vi "Cycle Diag Table Read.vi"(5 "Raw Data In":string) -> (4 "output cluster":T1)   [LabVIEW 2016, in "TLMB.lvlib"]
uses:
  Projects/TLMB.lvlib
  type defs/Cycle_Diag_Teststand.ctl
panel:
  out "appended array":string[](array[string])
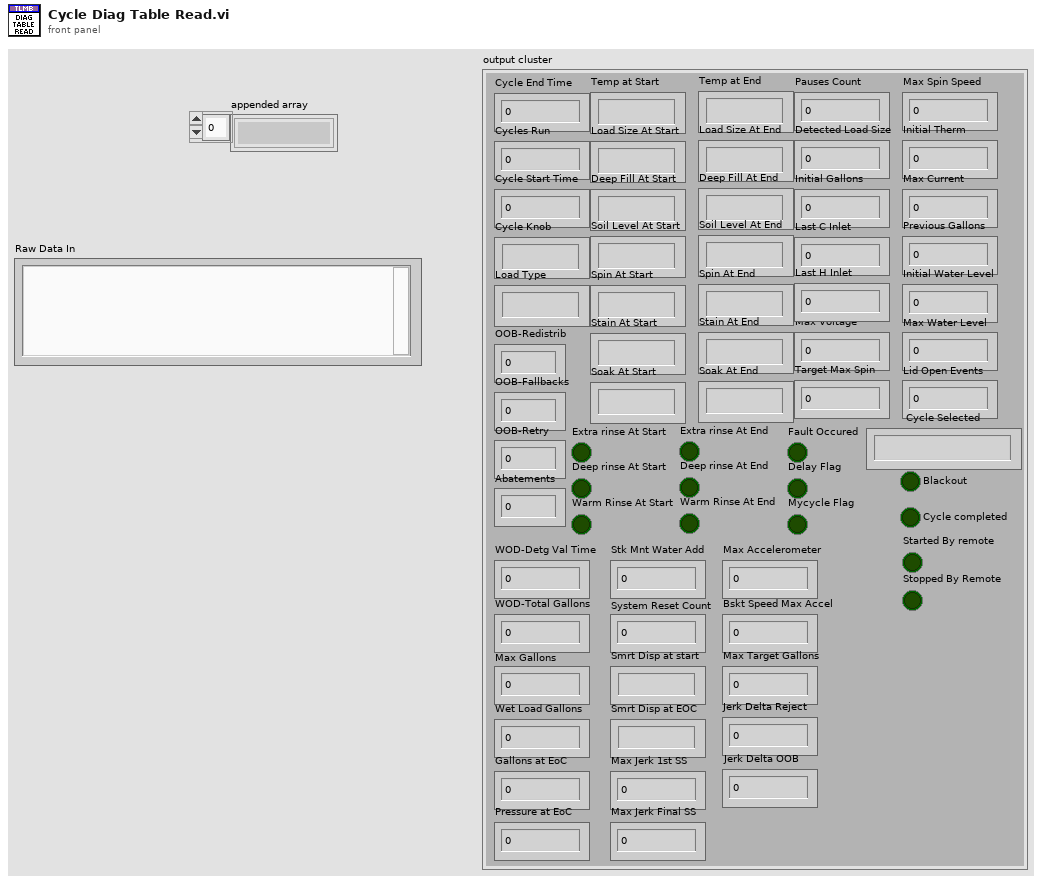
[diagram p1: front panel]
types:
  T1 = typedef "TLMB.lvlib/Cycle_Diag_Teststand.ctl" = cluster{"Cycle End Time":u32, "Cycles Run":u32, "Cycle Start Time":u32, "Cycle Knob":string, "Load Type":string, "OOB-Redistrib":u8, "OOB-Fallbacks":u8, "OOB-Retry":u8, "Temp at Start":string, "Load Size At Start":string, "Deep Fill At Start":string, "Soil Level At Start":string, "Spin At Start":string, "Extra rinse At Start":bool, "Deep rinse At Start":bool, "Stain At Start":string, "Soak At Start":string, "Warm Rinse At Start":bool, "Temp at End":string, "Load Size At End":string, "Deep Fill At End":string, "Soil Level At End":string, "Spin At End":string, "Extra rinse At End":bool, "Deep rinse At End":bool, "Stain At End":string, "Soak At End":string, "Warm Rinse At End":bool, "Pauses Count":u8, "Fault Occured":bool, "Delay Flag":bool, "Mycycle Flag":bool, "Blackout":bool, "Cycle completed":bool, "Detected Load Size":dbl, "Initial Gallons":dbl, "Last C Inlet ":dbl, "Max Voltage":dbl, "Target Max Spin":u16, "Max Spin Speed":u16, "Initial Therm":dbl, "Max Current":dbl, "Previous Gallons":dbl, "Initial Water Level":dbl, "Max Water Level":dbl, "Abatements ":u8, "Lid Open Events":u8, "Cycle Selected":string, "Last H Inlet ":dbl, "WOD-Detg Val Time":u8, "WOD-Total Gallons":u16, "Max Gallons":u16, "Wet Load Gallons":u16, "Gallons at EoC":u16, "Pressure at EoC":u32, "Stk Mnt Water Add":u8, "Started By remote":bool, "Stopped By Remote":bool, "System Reset Count":u8, "Smrt Disp at start":string, "Smrt Disp at EOC":string, "Max Jerk 1st SS":i32, "Max Jerk Final SS":i32, "Max Accelerometer":i16, "Bskt Speed Max Accel":u16, "Max Target Gallons":u16, "Jerk Delta Reject":u8, "Jerk Delta OOB ":u8}
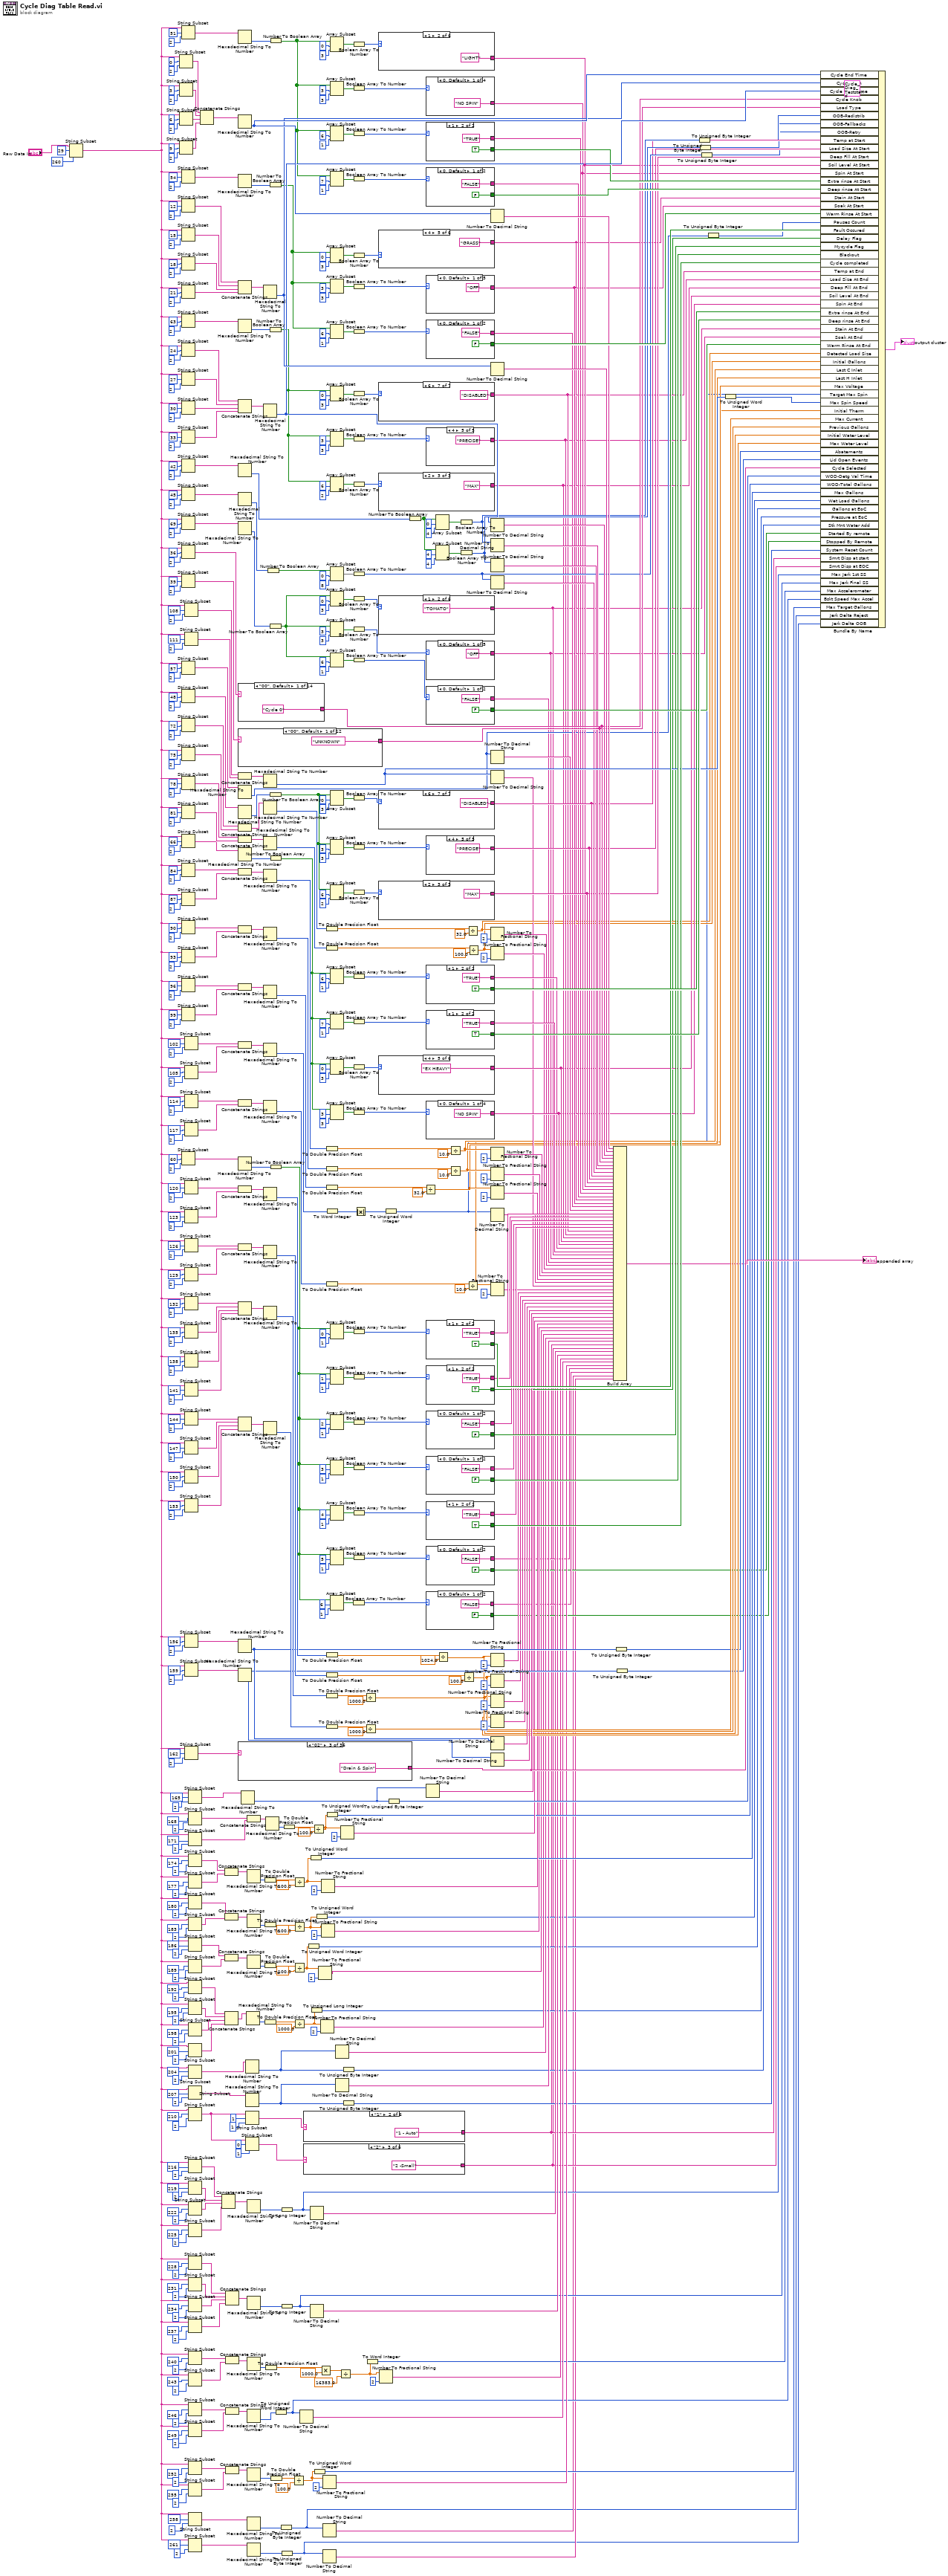
[diagram p0: block diagram]
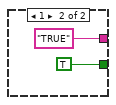
[diagram p2: hidden frame]
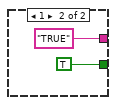
[diagram p3: hidden frame]
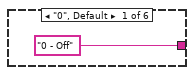
[diagram p4: hidden frame]
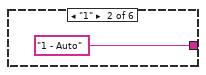
[diagram p5: hidden frame]
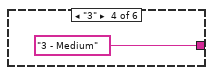
[diagram p6: hidden frame]
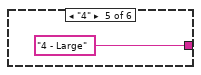
[diagram p7: hidden frame]
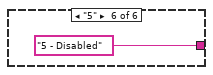
[diagram p8: hidden frame]
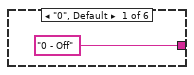
[diagram p9: hidden frame]
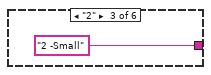
[diagram p10: hidden frame]
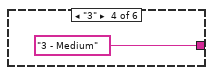
[diagram p11: hidden frame]
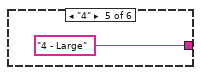
[diagram p12: hidden frame]
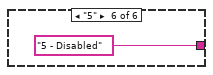
[diagram p13: hidden frame]
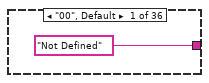
[diagram p14: hidden frame]
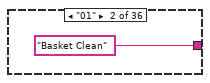
[diagram p15: hidden frame]
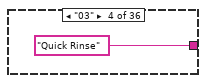
[diagram p16: hidden frame]
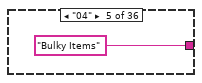
[diagram p17: hidden frame]
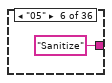
[diagram p18: hidden frame]
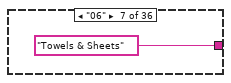
[diagram p19: hidden frame]
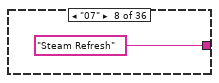
[diagram p20: hidden frame]
diagram:
  n1 = String Subset(string="Raw Data In", offset (0)=29, length (rest)=260 ("length (rest)")) -> (substring=w13:string)
  n2 = String Subset(string=w13, offset (0)=0, length (rest)=2 ("length (rest)")) -> (substring=w614:string)
  n3 = String Subset(string=w13, offset (0)=3, length (rest)=2 ("length (rest)")) -> (substring=w613:string)
  n4 = String Subset(string=w13, offset (0)=6, length (rest)=2 ("length (rest)")) -> (substring=w612:string)
  n5 = String Subset(string=w13, offset (0)=9, length (rest)=2 ("length (rest)")) -> (substring=w611:string)
  n6 = String Subset(string=w13, offset (0)=51, length (rest)=2 ("length (rest)")) -> (substring=w317:string)
  n7 = String Subset(string=w13, offset (0)=54, length (rest)=2 ("length (rest)")) -> (substring=w301:string)
  n8 = String Subset(string=w13, offset (0)=12, length (rest)=2 ("length (rest)")) -> (substring=w608:string)
  n9 = String Subset(string=w13, offset (0)=15, length (rest)=2 ("length (rest)")) -> (substring=w607:string)
  n10 = String Subset(string=w13, offset (0)=18, length (rest)=2 ("length (rest)")) -> (substring=w606:string)
  n11 = String Subset(string=w13, offset (0)=21, length (rest)=2 ("length (rest)")) -> (substring=w605:string)
  n12 = String Subset(string=w13, offset (0)=63, length (rest)=2 ("length (rest)")) -> (substring=w288:string)
  n13 = String Subset(string=w13, offset (0)=24, length (rest)=2 ("length (rest)")) -> (substring=w602:string)
  n14 = String Subset(string=w13, offset (0)=27, length (rest)=2 ("length (rest)")) -> (substring=w601:string)
  n15 = String Subset(string=w13, offset (0)=30, length (rest)=2 ("length (rest)")) -> (substring=w600:string)
  n16 = String Subset(string=w13, offset (0)=33, length (rest)=2 ("length (rest)")) -> (substring=w599:string)
  n17 = String Subset(string=w13, offset (0)=42, length (rest)=2 ("length (rest)")) -> (substring=w257:string)
  n18 = String Subset(string=w13, offset (0)=45, length (rest)=2 ("length (rest)")) -> (substring=w248:string)
  n19 = String Subset(string=w13, offset (0)=69, length (rest)=2 ("length (rest)")) -> (substring=w261:string)
  n20 = String Subset(string=w13, offset (0)=36, length (rest)=2 ("length (rest)")) -> (substring=w596:string)
  n21 = String Subset(string=w13, offset (0)=39, length (rest)=2 ("length (rest)")) -> (substring=w595:string)
  n22 = String Subset(string=w13, offset (0)=57, length (rest)=2 ("length (rest)")) -> (substring=w553:string)
  n23 = String Subset(string=w13, offset (0)=48, length (rest)=2 ("length (rest)")) -> (substring=w336:string)
  n24 = String Subset(string=w13, offset (0)=72, length (rest)=2 ("length (rest)")) -> (substring=w537:string)
  n25 = String Subset(string=w13, offset (0)=75 ("offset"), length (rest)=u32 2 ("default (0 U32)")) -> (substring=w534:string)
  n26 = String Subset(string=w13, offset (0)=78, length (rest)=2 ("length (rest)")) -> (substring=w529:string)
  n27 = String Subset(string=w13, offset (0)=81, length (rest)=2 ("length (rest)")) -> (substring=w528:string)
  n28 = String Subset(string=w13, offset (0)=66, length (rest)=2 ("length (rest)")) -> (substring=w274:string)
  n29 = String Subset(string=w13, offset (0)=84, length (rest)=2 ("length (rest)")) -> (substring=w518:string)
  n30 = String Subset(string=w13, offset (0)=87, length (rest)=2 ("length (rest)")) -> (substring=w517:string)
  n31 = String Subset(string=w13, offset (0)=90, length (rest)=2 ("length (rest)")) -> (substring=w512:string)
  n32 = String Subset(string=w13, offset (0)=93, length (rest)=2 ("length (rest)")) -> (substring=w511:string)
  n33 = String Subset(string=w13, offset (0)=96, length (rest)=2 ("length (rest)")) -> (substring=w502:string)
  n34 = String Subset(string=w13, offset (0)=99, length (rest)=2 ("length (rest)")) -> (substring=w501:string)
  n35 = String Subset(string=w13, offset (0)=60, length (rest)=2 ("length (rest)")) -> (substring=w552:string)
  n36 = String Subset(string=w13, offset (0)=108, length (rest)=2 ("length (rest)")) -> (substring=w489:string)
  n37 = String Subset(string=w13, offset (0)=111, length (rest)=2 ("length (rest)")) -> (substring=w488:string)
  n38 = String Subset(string=w13, offset (0)=102, length (rest)=2 ("length (rest)")) -> (substring=w492:string)
  n39 = String Subset(string=w13, offset (0)=105, length (rest)=2 ("length (rest)")) -> (substring=w491:string)
  n40 = String Subset(string=w13, offset (0)=114, length (rest)=2 ("length (rest)")) -> (substring=w477:string)
  n41 = String Subset(string=w13, offset (0)=117, length (rest)=2 ("length (rest)")) -> (substring=w476:string)
  n42 = String Subset(string=w13, offset (0)=120, length (rest)=2 ("length (rest)")) -> (substring=w467:string)
  n43 = String Subset(string=w13, offset (0)=123, length (rest)=2 ("length (rest)")) -> (substring=w466:string)
  n44 = String Subset(string=w13, offset (0)=126, length (rest)=2 ("length (rest)")) -> (substring=w457:string)
  n45 = String Subset(string=w13, offset (0)=129, length (rest)=2 ("length (rest)")) -> (substring=w456:string)
  n46 = String Subset(string=w13, offset (0)=132, length (rest)=2 ("length (rest)")) -> (substring=w447:string)
  n47 = String Subset(string=w13, offset (0)=135, length (rest)=2 ("length (rest)")) -> (substring=w446:string)
  n48 = String Subset(string=w13, offset (0)=138, length (rest)=2 ("length (rest)")) -> (substring=w416:string)
  n49 = String Subset(string=w13, offset (0)=141, length (rest)=2 ("length (rest)")) -> (substring=w415:string)
  n50 = String Subset(string=w13, offset (0)=144, length (rest)=2 ("length (rest)")) -> (substring=w441:string)
  n51 = String Subset(string=w13, offset (0)=147, length (rest)=2 ("length (rest)")) -> (substring=w440:string)
  n52 = String Subset(string=w13, offset (0)=150, length (rest)=2 ("length (rest)")) -> (substring=w410:string)
  n53 = String Subset(string=w13, offset (0)=153, length (rest)=2 ("length (rest)")) -> (substring=w409:string)
  n54 = String Subset(string=w13, offset (0)=156, length (rest)=2 ("length (rest)")) -> (substring=w421:string)
  n55 = String Subset(string=w13, offset (0)=159, length (rest)=2 ("length (rest)")) -> (substring=w420:string)
  n56 = String Subset(string=w13, offset (0)=162, length (rest)=2 ("length (rest)")) -> (substring=w417:string)
  n57 = String Subset(string=w13, offset (0)=165 ("length (rest)"), length (rest)=2 ("length (rest)")) -> (substring=w143:string)
  n58 = String Subset(string=w13, offset (0)=168 ("length (rest)"), length (rest)=2 ("length (rest)")) -> (substring=w141:string)
  n59 = String Subset(string=w13, offset (0)=171 ("length (rest)"), length (rest)=2 ("length (rest)")) -> (substring=w140:string)
  n60 = String Subset(string=w13, offset (0)=174 ("length (rest)"), length (rest)=2 ("length (rest)")) -> (substring=w131:string)
  n61 = String Subset(string=w13, offset (0)=177 ("length (rest)"), length (rest)=2 ("length (rest)")) -> (substring=w130:string)
  n62 = String Subset(string=w13, offset (0)=180 ("length (rest)"), length (rest)=2 ("length (rest)")) -> (substring=w121:string)
  n63 = String Subset(string=w13, offset (0)=183 ("length (rest)"), length (rest)=2 ("length (rest)")) -> (substring=w120:string)
  n64 = String Subset(string=w13, offset (0)=186 ("length (rest)"), length (rest)=2 ("length (rest)")) -> (substring=w119:string)
  n65 = String Subset(string=w13, offset (0)=189 ("length (rest)"), length (rest)=2 ("length (rest)")) -> (substring=w118:string)
  n66 = String Subset(string=w13, offset (0)=192 ("length (rest)"), length (rest)=2 ("length (rest)")) -> (substring=w117:string)
  n67 = String Subset(string=w13, offset (0)=195 ("length (rest)"), length (rest)=2 ("length (rest)")) -> (substring=w116:string)
  n68 = String Subset(string=w13, offset (0)=198 ("length (rest)"), length (rest)=2 ("length (rest)")) -> (substring=w115:string)
  n69 = String Subset(string=w13, offset (0)=201 ("length (rest)"), length (rest)=2 ("length (rest)")) -> (substring=w114:string)
  n70 = String Subset(string=w13, offset (0)=204 ("length (rest)"), length (rest)=2 ("length (rest)")) -> (substring=w109:string)
  n71 = String Subset(string=w13, offset (0)=207 ("length (rest)"), length (rest)=2 ("length (rest)")) -> (substring=w106:string)
  n72 = String Subset(string=w13, offset (0)=210 ("length (rest)"), length (rest)=2 ("length (rest)")) -> (substring=w105:string)
  n73 = String Subset(string=w13, offset (0)=216 ("length (rest)"), length (rest)=2 ("length (rest)")) -> (substring=w98:string)
  n74 = String Subset(string=w13, offset (0)=219 ("length (rest)"), length (rest)=2 ("length (rest)")) -> (substring=w97:string)
  n75 = String Subset(string=w13, offset (0)=222 ("length (rest)"), length (rest)=2 ("length (rest)")) -> (substring=w96:string)
  n76 = String Subset(string=w13, offset (0)=225 ("length (rest)"), length (rest)=2 ("length (rest)")) -> (substring=w95:string)
  n77 = String Subset(string=w13, offset (0)=228 ("length (rest)"), length (rest)=2 ("length (rest)")) -> (substring=w92:string)
  n78 = String Subset(string=w13, offset (0)=231 ("length (rest)"), length (rest)=2 ("length (rest)")) -> (substring=w91:string)
  n79 = String Subset(string=w13, offset (0)=234 ("length (rest)"), length (rest)=2 ("length (rest)")) -> (substring=w90:string)
  n80 = String Subset(string=w13, offset (0)=237 ("length (rest)"), length (rest)=2 ("length (rest)")) -> (substring=w89:string)
  n81 = String Subset(string=w13, offset (0)=240 ("length (rest)"), length (rest)=2 ("length (rest)")) -> (substring=w86:string)
  n82 = String Subset(string=w13, offset (0)=243 ("length (rest)"), length (rest)=2 ("length (rest)")) -> (substring=w85:string)
  n83 = String Subset(string=w13, offset (0)=246 ("length (rest)"), length (rest)=2 ("length (rest)")) -> (substring=w84:string)
  n84 = String Subset(string=w13, offset (0)=249 ("length (rest)"), length (rest)=2 ("length (rest)")) -> (substring=w83:string)
  n85 = String Subset(string=w13, offset (0)=252 ("length (rest)"), length (rest)=2 ("length (rest)")) -> (substring=w82:string)
  n86 = String Subset(string=w13, offset (0)=255 ("length (rest)"), length (rest)=2 ("length (rest)")) -> (substring=w81:string)
  n87 = String Subset(string=w13, offset (0)=258, length (rest)=2 ("length (rest)")) -> (substring=w8:string)
  n88 = String Subset(string=w13, offset (0)=261, length (rest)=2 ("length (rest)")) -> (substring=w7:string)
  n89 = Concatenate Strings(w614, w613, w612, w611) -> (w610:string)
  n90 = Concatenate Strings(w98, w97, w96, w95) -> (w94:string)
  n91 = Concatenate Strings(w131, w130) -> (w135:string)
  n92 = Concatenate Strings(w121, w120) -> (w129:string)
  n93 = Concatenate Strings(w119, w118) -> (w125:string)
  n94 = Concatenate Strings(w117, w116, w115, w114) -> (w110:string)
  n95 = Concatenate Strings(w92, w91, w90, w89) -> (w88:string)
  n96 = Concatenate Strings(w86, w85) -> (w79:string)
  n97 = Concatenate Strings(w84, w83) -> (w74:string)
  n98 = Concatenate Strings(w82, w81) -> (w72:string)
  n99 = Hexadecimal String To Number(string=w317) -> (number=w324:u32)  [unwired: 2 in, 1 out]
  n100 = Hexadecimal String To Number(string=w610) -> (number=w609:u32)  [unwired: 2 in, 1 out]
  n101 = Hexadecimal String To Number(string=w301) -> (number=w309:u32)  [unwired: 2 in, 1 out]
  n102 = Concatenate Strings(w608, w607, w606, w605) -> (w604:string)
  n103 = Hexadecimal String To Number(string=w288) -> (number=w296:u32)  [unwired: 2 in, 1 out]
  n104 = Concatenate Strings(w602, w601, w600, w599) -> (w598:string)
  n105 = Hexadecimal String To Number(string=w257) -> (number=w256:u32)  [unwired: 2 in, 1 out]
  n106 = Hexadecimal String To Number(string=w248) -> (number=w247:u32)  [unwired: 2 in, 1 out]
  n107 = Hexadecimal String To Number(string=w261) -> (number=w269:u32)  [unwired: 2 in, 1 out]
  n108 = case shown="\"00\", Default" w596 {
    tunnel: ["Cycle 0" "Cycle 1" "Cycle 2" "Cycle 3" "Cycle 4" "Cycle 5" "Cycle 6" "Cycle 7" "Cycle 8" "Cycle 9" "Cycle 10" "Cycle 11" "Cycle 12" "Cycle 13"] -> w397
    frame "00", Default {
    }
    frame "01" {
    }
    frame "02" {
    }
    frame "03" {
    }
    frame "04" {
    }
    frame "05" {
    }
    frame "06" {
    }
    frame "07" {
    }
    frame "08" {
    }
    frame "09" {
    }
    frame "0A" {
    }
    frame "0B" {
    }
    frame "0C" {
    }
    frame "0D" {
    }
  }
  n109 = case shown="\"00\", Default" w595 {
    tunnel: ["UNKNOWN" "COTTON" "SYNTHETIC" "MIXED" "WET" "LOW FLOW" "SMALL" "MEDIUM" "LARGE" "SUPER" "SUPER PLUS" "MAX"] -> w396
    frame "00", Default {
    }
    frame "01" {
    }
    frame "02" {
    }
    frame "03" {
    }
    frame "04" {
    }
    frame "05" {
    }
    frame "06" {
    }
    frame "07" {
    }
    frame "08" {
    }
    frame "09" {
    }
    frame "0A" {
    }
    frame "0B" {
    }
  }
  n110 = Concatenate Strings(w489, w488) -> (w487:string)
  n111 = Hexadecimal String To Number(string=w553) -> (number=w380:u32)  [unwired: 2 in, 1 out]
  n112 = Hexadecimal String To Number(string=w336) -> (number=w335:u32)  [unwired: 2 in, 1 out]
  n113 = Concatenate Strings(w537, w534) -> (w533:string)
  n114 = Concatenate Strings(w529, w528) -> (w527:string)
  n115 = Hexadecimal String To Number(string=w274) -> (number=w284:u32)  [unwired: 2 in, 1 out]
  n116 = Concatenate Strings(w518, w517) -> (w516:string)
  n117 = Concatenate Strings(w512, w511) -> (w510:string)
  n118 = Concatenate Strings(w502, w501) -> (w500:string)
  n119 = Concatenate Strings(w492, w491) -> (w490:string)
  n120 = Concatenate Strings(w477, w476) -> (w475:string)
  n121 = Hexadecimal String To Number(string=w552) -> (number=w551:u32)  [unwired: 2 in, 1 out]
  n122 = Concatenate Strings(w467, w466) -> (w465:string)
  n123 = Concatenate Strings(w457, w456) -> (w455:string)
  n124 = Concatenate Strings(w447, w446, w416, w415) -> (w445:string)
  n125 = Concatenate Strings(w441, w440, w410, w409) -> (w439:string)
  n126 = Hexadecimal String To Number(string=w421) -> (number=w419:u32)  [unwired: 2 in, 1 out]
  n127 = Hexadecimal String To Number(string=w420) -> (number=w418:u32)  [unwired: 2 in, 1 out]
  n128 = case shown="\"02\"" w417 {
    tunnel: ["Not Defined" "Basket Clean" "Drain & Spin" "Quick Rinse" "Bulky Items" "Sanitize" "Towels & Sheets" "Steam Refresh" "Normal/Mixed" "Whites" "Dark Colors" "Jeans" "Hand Wash" "Delicates" "Speed Wash" "Heavy Duty" "Allergen" "Power Clean" "Rinse & Spin" "Single Item" "Colors" "Cold Wash" "Cottons" "Easy Care" "Active Wear" "Timed Dry" "Dewrinkle" "Air Fluff" "Steam Refresh" "Steam Dewrinkle" "Speed Dry" "Mixed" "Quick Dry" "Casuals" "Warm Up" "Energy Saver"] -> w347
    frame "00", Default {
    }
    frame "01" {
    }
    frame "02" {
    }
    frame "03" {
    }
    frame "04" {
    }
    frame "05" {
    }
    frame "06" {
    }
    frame "07" {
    }
    frame "08" {
    }
    frame "09" {
    }
    frame "0A" {
    }
    frame "0B" {
    }
    frame "0C" {
    }
    frame "0D" {
    }
    frame "0E" {
    }
    frame "0F" {
    }
    frame "10" {
    }
    frame "11" {
    }
    frame "12" {
    }
    frame "13" {
    }
    frame "14" {
    }
    frame "15" {
    }
    frame "80" {
    }
    frame "81" {
    }
    frame "82" {
    }
    frame "83" {
    }
    frame "84" {
    }
    frame "85" {
    }
    frame "86" {
    }
    frame "87" {
    }
    frame "88" {
    }
    frame "89" {
    }
    frame "8A" {
    }
    frame "8B" {
    }
    frame "8C" {
    }
    frame "8D" {
    }
  }
  n129 = Hexadecimal String To Number(string=w143) -> (number=w142:u32)  [unwired: 2 in, 1 out]
  n130 = Hexadecimal String To Number(string=w109) -> (number=w108:u32)  [unwired: 2 in, 1 out]
  n131 = Hexadecimal String To Number(string=w106) -> (number=w107:u32)  [unwired: 2 in, 1 out]
  n132 = String Subset(string=w105, offset (0)=1, length (rest)=1 ("length (rest)")) -> (substring=w100:string)
  n133 = String Subset(string=w105, offset (0)=0, length (rest)=1 ("length (rest)")) -> (substring=w99:string)
  n134 = Hexadecimal String To Number(string=w110) -> (number=w113:u32)  [unwired: 2 in, 1 out]
  n135 = Concatenate Strings(w141, w140) -> (w139:string)
  n136 = Hexadecimal String To Number(string=w135) -> (number=w134:u32)  [unwired: 2 in, 1 out]
  n137 = Hexadecimal String To Number(string=w129) -> (number=w128:u32)  [unwired: 2 in, 1 out]
  n138 = Hexadecimal String To Number(string=w125) -> (number=w124:u32)  [unwired: 2 in, 1 out]
  n139 = Hexadecimal String To Number(string=w79) -> (number=w80:u32)  [unwired: 2 in, 1 out]
  n140 = Hexadecimal String To Number(string=w74) -> (number=w55:u32)  [unwired: 2 in, 1 out]
  n141 = Hexadecimal String To Number(string=w72) -> (number=w73:u32)  [unwired: 2 in, 1 out]
  n142 = Hexadecimal String To Number(string=w8) -> (number=w6:u32)  [unwired: 2 in, 1 out]
  n143 = Hexadecimal String To Number(string=w7) -> (number=w5:u32)  [unwired: 2 in, 1 out]
  n144 = Hexadecimal String To Number(string=w94) -> (number=w93:u32)  [unwired: 2 in, 1 out]
  n145 = Hexadecimal String To Number(string=w88) -> (number=w87:u32)  [unwired: 2 in, 1 out]
  n146 = Hexadecimal String To Number(string=w604) -> (number=w603:u32)  [unwired: 2 in, 1 out]
  n147 = Hexadecimal String To Number(string=w598) -> (number=w597:u32)  [unwired: 2 in, 1 out]
  n148 = Hexadecimal String To Number(string=w487) -> (number=w486:u32)  [unwired: 2 in, 1 out]
  n149 = Hexadecimal String To Number(string=w533) -> (number=w540:u32)  [unwired: 2 in, 1 out]
  n150 = Hexadecimal String To Number(string=w527) -> (number=w526:u32)  [unwired: 2 in, 1 out]
  n151 = Hexadecimal String To Number(string=w516) -> (number=w515:u32)  [unwired: 2 in, 1 out]
  n152 = Hexadecimal String To Number(string=w510) -> (number=w509:u32)  [unwired: 2 in, 1 out]
  n153 = Hexadecimal String To Number(string=w500) -> (number=w499:u32)  [unwired: 2 in, 1 out]
  n154 = Hexadecimal String To Number(string=w490) -> (number=w402:u32)  [unwired: 2 in, 1 out]
  n155 = Hexadecimal String To Number(string=w475) -> (number=w474:u32)  [unwired: 2 in, 1 out]
  n156 = Hexadecimal String To Number(string=w465) -> (number=w464:u32)  [unwired: 2 in, 1 out]
  n157 = Hexadecimal String To Number(string=w455) -> (number=w454:u32)  [unwired: 2 in, 1 out]
  n158 = Hexadecimal String To Number(string=w445) -> (number=w444:u32)  [unwired: 2 in, 1 out]
  n159 = Hexadecimal String To Number(string=w439) -> (number=w438:u32)  [unwired: 2 in, 1 out]
  n160 = To Double Precision Float(number=w134) -> (double precision float=w133:dbl)
  n161 = To Double Precision Float(number=w128) -> (double precision float=w127:dbl)
  n162 = To Double Precision Float(number=w124) -> (double precision float=w123:dbl)
  n163 = To Double Precision Float(number=w113) -> (double precision float=w112:dbl)
  n164 = To Double Precision Float(number=w80) -> (double precision float=w78:dbl)
  n165 = Hexadecimal String To Number(string=w139) -> (number=w138:u32)  [unwired: 2 in, 1 out]
  n166 = Number To Boolean Array(number=w247) -> (Boolean array=w246:bool[])
  n167 = Number To Boolean Array(number=w309) -> (Boolean array=w308:bool[])
  n168 = Number To Boolean Array(number=w296) -> (Boolean array=w295:bool[])
  n169 = Number To Boolean Array(number=w269) -> (Boolean array=w268:bool[])
  n170 = Number To Boolean Array(number=w335) -> (Boolean array=w334:bool[])
  n171 = Number To Boolean Array(number=w324) -> (Boolean array=w316:bool[])
  n172 = Number To Boolean Array(number=w284) -> (Boolean array=w277:bool[])
  n173 = Number To Boolean Array(number=w551) -> (Boolean array=w30:bool[])
  n174 = To Double Precision Float(number=w73) -> (double precision float=w71:dbl)
  n175 = To Unsigned Word Integer(number=w55) -> (unsigned 16bit integer=w15:u16)
  n176 = To Unsigned Byte Integer(number=w6) -> (unsigned 8bit integer=w2:u8)
  n177 = To Long Integer(number=w93) -> (32bit integer=w18:i32)
  n178 = To Long Integer(number=w87) -> (32bit integer=w17:i32)
  n179 = To Unsigned Byte Integer(number=w5) -> (unsigned 8bit integer=w1:u8)
  n180 = To Double Precision Float(number=w138) -> (double precision float=w137:dbl)
  n181 = Divide(x=w71, y=100.0) -> (x/y=w63:dbl)
  n182 = Divide(x=w133, y=100.0) -> (x/y=w68:dbl)
  n183 = Divide(x=w127, y=100.0) -> (x/y=w67:dbl)
  n184 = Divide(x=w123, y=100.0) -> (x/y=w66:dbl)
  n185 = Divide(x=w112, y=1000.0) -> (x/y=w65:dbl)
  n186 = Number To Decimal String(number=w15) -> (decimal integer string=w40:string)  [unwired: 1 in]
  n187 = case shown="\"2\"" w99 {
    tunnel: ["0 - Off" "1 - Auto" "2 -Small" "3 - Medium" "4 - Large" "5 - Disabled"] -> w19
    frame "0", Default {
    }
    frame "1" {
    }
    frame "2" {
    }
    frame "3" {
    }
    frame "4" {
    }
    frame "5" {
    }
  }
  n188 = case shown="\"1\"" w100 {
    tunnel: ["0 - Off" "1 - Auto" "2 -Small" "3 - Medium" "4 - Large" "5 - Disabled"] -> w20
    frame "0", Default {
    }
    frame "1" {
    }
    frame "2" {
    }
    frame "3" {
    }
    frame "4" {
    }
    frame "5" {
    }
  }
  n189 = To Unsigned Word Integer(number=w66) -> (unsigned 16bit integer=w26:u16)
  n190 = To Unsigned Word Integer(number=w68) -> (unsigned 16bit integer=w49:u16)
  n191 = To Unsigned Long Integer(number=w65) -> (unsigned 32bit integer=w25:u32)
  n192 = Number To Decimal String(number=w18) -> (decimal integer string=w43:string)  [unwired: 1 in]
  n193 = Number To Decimal String(number=w17) -> (decimal integer string=w42:string)  [unwired: 1 in]
  n194 = Divide(x=w137, y=100.0) -> (x/y=w69:dbl)
  n195 = To Unsigned Word Integer(number=w63) -> (unsigned 16bit integer=w14:u16)
  n196 = To Unsigned Word Integer(number=w67) -> (unsigned 16bit integer=w27:u16)
  n197 = Number To Fractional String(number=w66, precision (6)=i16 2) -> (F-format string=w47:string)  [unwired: 2 in]
  n198 = Multiply(x=w78, y=1000.0) -> (x*y=w76:dbl)
  n199 = Number To Fractional String(number=w65, precision (6)=i16 2) -> (F-format string=w46:string)  [unwired: 2 in]
  n200 = Number To Fractional String(number=w68, precision (6)=i16 2) -> (F-format string=w50:string)  [unwired: 2 in]
  n201 = Number To Fractional String(number=w67, precision (6)=i16 2) -> (F-format string=w48:string)  [unwired: 2 in]
  n202 = Number To Fractional String(number=w63, precision (6)=i16 2) -> (F-format string=w39:string)  [unwired: 2 in]
  n203 = Number To Decimal String(number=w2) -> (decimal integer string=w4:string)  [unwired: 1 in]
  n204 = Number To Decimal String(number=w1) -> (decimal integer string=w3:string)  [unwired: 1 in]
  n205 = To Double Precision Float(number=w540) -> (double precision float=w539:dbl)
  n206 = To Double Precision Float(number=w526) -> (double precision float=w525:dbl)
  n207 = To Double Precision Float(number=w515) -> (double precision float=w514:dbl)
  n208 = To Double Precision Float(number=w509) -> (double precision float=w508:dbl)
  n209 = To Double Precision Float(number=w499) -> (double precision float=w498:dbl)
  n210 = To Word Integer(number=w402) -> (16bit integer=w404:i16)
  n211 = To Double Precision Float(number=w474) -> (double precision float=w473:dbl)
  n212 = To Double Precision Float(number=w464) -> (double precision float=w463:dbl)
  n213 = To Double Precision Float(number=w454) -> (double precision float=w453:dbl)
  n214 = To Double Precision Float(number=w444) -> (double precision float=w443:dbl)
  n215 = To Double Precision Float(number=w438) -> (double precision float=w437:dbl)
  n216 = To Unsigned Word Integer(number=w69) -> (unsigned 16bit integer=w51:u16)
  n217 = Array Subset(array=w30, index=6, length=1) -> (w31:bool[])
  n218 = Array Subset(array=w316, index=0, length=3) -> (w313:bool[])
  n219 = Array Subset(array=w316, index=3, length=3) -> (w312:bool[])
  n220 = Array Subset(array=w316, index=6, length=1) -> (w311:bool[])
  n221 = Array Subset(array=w316, index=7, length=1) -> (w310:bool[])
  n222 = Array Subset(array=w308, index=0, length=3) -> (w299:bool[])
  n223 = Array Subset(array=w308, index=3, length=3) -> (w298:bool[])
  n224 = Array Subset(array=w308, index=6, length=1) -> (w297:bool[])
  n225 = Array Subset(array=w295, index=0, length=3) -> (w287:bool[])
  n226 = Array Subset(array=w295, index=3, length=3) -> (w286:bool[])
  n227 = Array Subset(array=w295, index=6, length=2) -> (w285:bool[])
  n228 = Array Subset(array=w246, index=0, length=8) -> (w243:bool[])
  n229 = Array Subset(array=w268, index=0, length=3) -> (w260:bool[])
  n230 = Array Subset(array=w268, index=3, length=3) -> (w259:bool[])
  n231 = Array Subset(array=w268, index=6, length=1) -> (w258:bool[])
  n232 = Array Subset(array=w334, index=0, length=3) -> (w327:bool[])
  n233 = Array Subset(array=w334, index=3, length=3) -> (w326:bool[])
  n234 = Array Subset(array=w334, index=6, length=2) -> (w325:bool[])
  n235 = Array Subset(array=w277, index=6, length=1) -> (w271:bool[])
  n236 = Array Subset(array=w277, index=7, length=1) -> (w270:bool[])
  n237 = Array Subset(array=w277, index=0, length=3) -> (w273:bool[])
  n238 = Array Subset(array=w277, index=3, length=3) -> (w272:bool[])
  n239 = Array Subset(array=w30, index=0, length=1) -> (w232:bool[])
  n240 = Array Subset(array=w30, index=1, length=1) -> (w230:bool[])
  n241 = Array Subset(array=w30, index=2, length=1) -> (w229:bool[])
  n242 = Array Subset(array=w30, index=3, length=1) -> (w228:bool[])
  n243 = Array Subset(array=w30, index=4, length=1) -> (w227:bool[])
  n244 = Array Subset(array=w30, index=5, length=1) -> (w35:bool[])
  n245 = Number To Decimal String(number=w108) -> (decimal integer string=w45:string)  [unwired: 1 in]
  n246 = Number To Decimal String(number=w107) -> (decimal integer string=w44:string)  [unwired: 1 in]
  n247 = Divide(x=w76, y=16383.0) -> (x/y=w64:dbl)
  n248 = Number To Fractional String(number=w69, precision (6)=i16 2) -> (F-format string=w52:string)  [unwired: 2 in]
  n249 = To Unsigned Byte Integer(number=w108) -> (unsigned 8bit integer=w24:u8)
  n250 = To Unsigned Byte Integer(number=w107) -> (unsigned 8bit integer=w21:u8)
  n251 = Boolean Array To Number(Boolean array=w31) -> (number=w34:u32)
  n252 = Boolean Array To Number(Boolean array=w313) -> (number=w586:u32)
  n253 = Boolean Array To Number(Boolean array=w312) -> (number=w585:u32)
  n254 = Boolean Array To Number(Boolean array=w311) -> (number=w584:u32)
  n255 = Boolean Array To Number(Boolean array=w310) -> (number=w583:u32)
  n256 = Boolean Array To Number(Boolean array=w299) -> (number=w580:u32)
  n257 = Boolean Array To Number(Boolean array=w298) -> (number=w579:u32)
  n258 = Boolean Array To Number(Boolean array=w297) -> (number=w578:u32)
  n259 = Boolean Array To Number(Boolean array=w287) -> (number=w570:u32)
  n260 = Boolean Array To Number(Boolean array=w286) -> (number=w569:u32)
  n261 = Boolean Array To Number(Boolean array=w285) -> (number=w568:u32)
  n262 = Boolean Array To Number(Boolean array=w243) -> (number=w390:u32)
  n263 = Boolean Array To Number(Boolean array=w260) -> (number=w563:u32)
  n264 = Boolean Array To Number(Boolean array=w259) -> (number=w562:u32)
  n265 = Boolean Array To Number(Boolean array=w258) -> (number=w561:u32)
  n266 = Boolean Array To Number(Boolean array=w327) -> (number=w401:u32)
  n267 = Boolean Array To Number(Boolean array=w326) -> (number=w588:u32)
  n268 = Boolean Array To Number(Boolean array=w325) -> (number=w587:u32)
  n269 = Boolean Array To Number(Boolean array=w271) -> (number=w565:u32)
  n270 = Boolean Array To Number(Boolean array=w270) -> (number=w564:u32)
  n271 = Boolean Array To Number(Boolean array=w273) -> (number=w567:u32)
  n272 = Boolean Array To Number(Boolean array=w272) -> (number=w566:u32)
  n273 = Boolean Array To Number(Boolean array=w232) -> (number=w550:u32)
  n274 = Boolean Array To Number(Boolean array=w230) -> (number=w549:u32)
  n275 = Boolean Array To Number(Boolean array=w229) -> (number=w548:u32)
  n276 = Boolean Array To Number(Boolean array=w228) -> (number=w547:u32)
  n277 = Boolean Array To Number(Boolean array=w227) -> (number=w546:u32)
  n278 = Boolean Array To Number(Boolean array=w35) -> (number=w38:u32)
  n279 = Absolute Value(x=w404) -> (abs(x)=w403:i16)
  n280 = Divide(x=w443, y=1000.0) -> (x/y=w340:dbl)
  n281 = Divide(x=w437, y=1000.0) -> (x/y=w339:dbl)
  n282 = To Word Integer(number=w64) -> (16bit integer=w16:i16)
  n283 = case shown="1" w586 {
    tunnel: ["EXTRA LIGHT" "LIGHT" "NORMAL" "HEAVY" "EX HEAVY" "DISABLED"] -> w386
    frame 0, Default {
    }
    frame 1 {
    }
    frame 2 {
    }
    frame 3 {
    }
    frame 4 {
    }
    frame 5 {
    }
  }
  n284 = case shown="4" w580 {
    tunnel: ["OFF" "TOMATO" "WINE" "BLOOD" "GRASS" "DIRT"] -> w300
    frame 0, Default {
    }
    frame 1 {
    }
    frame 2 {
    }
    frame 3 {
    }
    frame 4 {
    }
    frame 5 {
    }
  }
  n285 = case shown="6" w570 {
    tunnel: ["TAP COLD" "COLD" "COOL" "COLORS" "WARM" "HOT" "DISABLED"] -> w372
    frame 0, Default {
    }
    frame 1 {
    }
    frame 2 {
    }
    frame 3 {
    }
    frame 4 {
    }
    frame 5 {
    }
    frame 6 {
    }
  }
  n286 = case shown="2" w568 {
    tunnel: ["OFF" "INCREMENTAL" "MAX"] -> w370
    frame 0, Default {
    }
    frame 1 {
    }
    frame 2 {
    }
  }
  n287 = case shown="1" w563 {
    tunnel: ["OFF" "TOMATO" "WINE" "BLOOD" "GRASS" "DIRT"] -> w365
    frame 0, Default {
    }
    frame 1 {
    }
    frame 2 {
    }
    frame 3 {
    }
    frame 4 {
    }
    frame 5 {
    }
  }
  n288 = case shown="6" w401 {
    tunnel: ["TAP COLD" "COLD" "COOL" "COLORS" "WARM" "HOT" "DISABLED"] -> w389
    frame 0, Default {
    }
    frame 1 {
    }
    frame 2 {
    }
    frame 3 {
    }
    frame 4 {
    }
    frame 5 {
    }
    frame 6 {
    }
  }
  n289 = case shown="2" w587 {
    tunnel: ["OFF" "INCREMENTAL" "MAX"] -> w387
    frame 0, Default {
    }
    frame 1 {
    }
    frame 2 {
    }
  }
  n290 = case shown="4" w567 {
    tunnel: ["EXTRA LIGHT" "LIGHT" "NORMAL" "HEAVY" "EX HEAVY" "DISABLED"] -> w369
    frame 0, Default {
    }
    frame 1 {
    }
    frame 2 {
    }
    frame 3 {
    }
    frame 4 {
    }
    frame 5 {
    }
  }
  n291 = Number To Fractional String(number=w64, precision (6)=i16 2) -> (F-format string=w41:string)  [unwired: 2 in]
  n292 = To Unsigned Word Integer(number=w403) -> (unsigned 16bit integer=w216:u16)
  n293 = To Unsigned Byte Integer(number=w142) -> (unsigned 8bit integer=w53:u8)
  n294 = Number To Boolean Array(number=w256) -> (Boolean array=w251:bool[])
  n295 = Divide(x=w498, y=32.0) -> (x/y=w344:dbl)
  n296 = case shown="0, Default" w34 {
    tunnel: [FALSE TRUE] -> w22
    tunnel: ["FALSE" "TRUE"] -> w28
    frame 0, Default {
    }
    frame 1 {
    }
  }
  n297 = case shown="0, Default" w585 {
    tunnel: ["NO SPIN" "NORMAL" "MORE" "MAX"] -> w385
    frame 0, Default {
    }
    frame 1 {
    }
    frame 2 {
    }
    frame 3 {
    }
  }
  n298 = case shown="1" w584 {
    tunnel: [FALSE TRUE] -> w582
    tunnel: ["FALSE" "TRUE"] -> w384
    frame 0, Default {
    }
    frame 1 {
    }
  }
  n299 = case shown="0, Default" w583 {
    tunnel: [FALSE TRUE] -> w581
    tunnel: ["FALSE" "TRUE"] -> w383
    frame 0, Default {
    }
    frame 1 {
    }
  }
  n300 = case shown="0, Default" w579 {
    tunnel: ["OFF" "15 MIN" "30 MIN" "60 MIN" "2 HOURS"] -> w382
    frame 0, Default {
    }
    frame 1 {
    }
    frame 2 {
    }
    frame 3 {
    }
    frame 4 {
    }
  }
  n301 = case shown="0, Default" w578 {
    tunnel: [FALSE TRUE] -> w577
    tunnel: ["FALSE" "TRUE"] -> w381
    frame 0, Default {
    }
    frame 1 {
    }
  }
  n302 = case shown="4" w569 {
    tunnel: ["SMALL" "MEDIUM" "LARGE" "SUPER" "PRECISE"] -> w371
    frame 0, Default {
    }
    frame 1 {
    }
    frame 2 {
    }
    frame 3 {
    }
    frame 4 {
    }
  }
  n303 = case shown="0, Default" w562 {
    tunnel: ["OFF" "15 MIN" "30 MIN" "60 MIN" "2 HOURS"] -> w364
    frame 0, Default {
    }
    frame 1 {
    }
    frame 2 {
    }
    frame 3 {
    }
    frame 4 {
    }
  }
  n304 = case shown="0, Default" w561 {
    tunnel: [FALSE TRUE] -> w558
    tunnel: ["FALSE" "TRUE"] -> w363
    frame 0, Default {
    }
    frame 1 {
    }
  }
  n305 = case shown="4" w588 {
    tunnel: ["SMALL" "MEDIUM" "LARGE" "SUPER" "PRECISE"] -> w388
    frame 0, Default {
    }
    frame 1 {
    }
    frame 2 {
    }
    frame 3 {
    }
    frame 4 {
    }
  }
  n306 = case shown="1" w565 {
    tunnel: [FALSE TRUE] -> w560
    tunnel: ["FALSE" "TRUE"] -> w367
    frame 0, Default {
    }
    frame 1 {
    }
  }
  n307 = case shown="1" w564 {
    tunnel: [FALSE TRUE] -> w559
    tunnel: ["FALSE" "TRUE"] -> w366
    frame 0, Default {
    }
    frame 1 {
    }
  }
  n308 = case shown="0, Default" w566 {
    tunnel: ["NO SPIN" "NORMAL" "MORE" "MAX"] -> w368
    frame 0, Default {
    }
    frame 1 {
    }
    frame 2 {
    }
    frame 3 {
    }
  }
  n309 = case shown="1" w550 {
    tunnel: [FALSE TRUE] -> w545
    tunnel: ["FALSE" "TRUE"] -> w377
    frame 0, Default {
    }
    frame 1 {
    }
  }
  n310 = case shown="1" w549 {
    tunnel: [FALSE TRUE] -> w231
    tunnel: ["FALSE" "TRUE"] -> w376
    frame 0, Default {
    }
    frame 1 {
    }
  }
  n311 = case shown="0, Default" w548 {
    tunnel: [FALSE TRUE] -> w378
    tunnel: ["FALSE" "TRUE"] -> w375
    frame 0, Default {
    }
    frame 1 {
    }
  }
  n312 = case shown="0, Default" w547 {
    tunnel: [FALSE TRUE] -> w544
    tunnel: ["FALSE" "TRUE"] -> w374
    frame 0, Default {
    }
    frame 1 {
    }
  }
  n313 = case shown="1" w546 {
    tunnel: [FALSE TRUE] -> w543
    tunnel: ["FALSE" "TRUE"] -> w373
    frame 0, Default {
    }
    frame 1 {
    }
  }
  n314 = case shown="0, Default" w38 {
    tunnel: [FALSE TRUE] -> w23
    tunnel: ["FALSE" "TRUE"] -> w29
    frame 0, Default {
    }
    frame 1 {
    }
  }
  n315 = Number To Decimal String(number=w142) -> (decimal integer string=w54:string)  [unwired: 1 in]
  n316 = Array Subset(array=w251, index=0, length=4) -> (w250:bool[])
  n317 = Array Subset(array=w251, index=4, length=4) -> (w249:bool[])
  n318 = Divide(x=w463, y=1024.0) -> (x/y=w342:dbl)
  n319 = Divide(x=w514, y=10.0) -> (x/y=w346:dbl)
  n320 = Divide(x=w508, y=10.0) -> (x/y=w345:dbl)
  n321 = Boolean Array To Number(Boolean array=w250) -> (number=w395:u32)
  n322 = Boolean Array To Number(Boolean array=w249) -> (number=w393:u32)
  n323 = Divide(x=w453, y=100.0) -> (x/y=w341:dbl)
  n324 = Divide(x=w539, y=32.0) -> (x/y=w362:dbl)
  n325 = Divide(x=w473, y=10.0) -> (x/y=w343:dbl)
  n326 = Divide(x=w525, y=100.0) -> (x/y=w338:dbl)
  n327 = Number To Decimal String(number=w609) -> (decimal integer string=w400:string)  [unwired: 1 in]
  n328 = Number To Decimal String(number=w603) -> (decimal integer string=w399:string)  [unwired: 1 in]
  n329 = Number To Decimal String(number=w597) -> (decimal integer string=w398:string)  [unwired: 1 in]
  n330 = Number To Decimal String(number=w395) -> (decimal integer string=w394:string)  [unwired: 1 in]
  n331 = Number To Decimal String(number=w393) -> (decimal integer string=w392:string)  [unwired: 1 in]
  n332 = Number To Decimal String(number=w390) -> (decimal integer string=w391:string)  [unwired: 1 in]
  n333 = Number To Decimal String(number=w380) -> (decimal integer string=w379:string)  [unwired: 1 in]
  n334 = Number To Decimal String(number=w486) -> (decimal integer string=w355:string)  [unwired: 1 in]
  n335 = Number To Fractional String(number=w362, precision (6)=i16 2) -> (F-format string=w361:string)  [unwired: 2 in]
  n336 = Number To Fractional String(number=w338, precision (6)=i16 2) -> (F-format string=w360:string)  [unwired: 2 in]
  n337 = Number To Fractional String(number=w346, precision (6)=i16 2) -> (F-format string=w359:string)  [unwired: 2 in]
  n338 = Number To Fractional String(number=w345, precision (6)=i16 2) -> (F-format string=w358:string)  [unwired: 2 in]
  n339 = Number To Fractional String(number=w344, precision (6)=i16 2) -> (F-format string=w357:string)  [unwired: 2 in]
  n340 = Number To Decimal String(number=w216) -> (decimal integer string=w356:string)  [unwired: 1 in]
  n341 = Number To Fractional String(number=w343, precision (6)=i16 2) -> (F-format string=w354:string)  [unwired: 2 in]
  n342 = Number To Fractional String(number=w342, precision (6)=i16 2) -> (F-format string=w353:string)  [unwired: 2 in]
  n343 = Number To Fractional String(number=w341, precision (6)=i16 2) -> (F-format string=w352:string)  [unwired: 2 in]
  n344 = Number To Fractional String(number=w340, precision (6)=i16 2) -> (F-format string=w351:string)  [unwired: 2 in]
  n345 = Number To Fractional String(number=w339, precision (6)=i16 2) -> (F-format string=w350:string)  [unwired: 2 in]
  n346 = Number To Decimal String(number=w419) -> (decimal integer string=w349:string)  [unwired: 1 in]
  n347 = Number To Decimal String(number=w418) -> (decimal integer string=w348:string)  [unwired: 1 in]
  n348 = Build Array(w400, w399, w398, w397, w396, w394, w392, w391, w389, w388, w387, w386, w385, w384, w383, w300, w382, w381, w379, w377, w376, w375, w374, w373, w372, w371, w370, w369, w368, w367, w366, w365, w364, w363, w361, w360, w359, w358, w357, w356, w355, w354, w353, w352, w351, w350, w349, w348, w347, w54, w52, w50, w48, w47, w46, w45, w44, w20, w19, w43, w42, w41, w40, w39, w29, w28, w4, w3) -> (→"appended array":string[])
  n349 = To Unsigned Byte Integer(number=w419) -> (unsigned 8bit integer=w215:u8)
  n350 = To Unsigned Byte Integer(number=w418) -> (unsigned 8bit integer=w214:u8)
  n351 = To Unsigned Byte Integer(number=w395) -> (unsigned 8bit integer=w226:u8)
  n352 = To Unsigned Byte Integer(number=w393) -> (unsigned 8bit integer=w225:u8)
  n353 = To Unsigned Byte Integer(number=w390) -> (unsigned 8bit integer=w224:u8)
  n354 = To Unsigned Byte Integer(number=w380) -> (unsigned 8bit integer=w223:u8)
  n355 = To Unsigned Word Integer(number=w486) -> (unsigned 16bit integer=w217:u16)
  n356 = Bundle By Name(cluster=T1 {"Cycle End Time"=0, "Cycles Run"=0, "Cycle Start Time"=0, "Cycle Knob"="", "Load Type"="", "OOB-Redistrib"=0, "OOB-Fallbacks"=0, "OOB-Retry"=0, "Temp at Start"="", "Load Size At Start"="", "Deep Fill At Start"="", "Soil Level At Start"="", "Spin At Start"="", "Extra rinse At Start"=FALSE, "Deep rinse At Start"=FALSE, "Stain At Start"="", "Soak At Start"="", "Warm Rinse At Start"=FALSE, "Temp at End"="", "Load Size At End"="", "Deep Fill At End"="", "Soil Level At End"="", "Spin At End"="", "Extra rinse At End"=FALSE, "Deep rinse At End"=FALSE, "Stain At End"="", "Soak At End"="", "Warm Rinse At End"=FALSE, "Pauses Count"=0, "Fault Occured"=FALSE, "Delay Flag"=FALSE, "Mycycle Flag"=FALSE, "Blackout"=FALSE, "Cycle completed"=FALSE, "Detected Load Size"=0.0, "Initial Gallons"=0.0, "Last C Inlet "=0.0, "Max Voltage"=0.0, "Target Max Spin"=0, "Max Spin Speed"=0, "Initial Therm"=0.0, "Max Current"=0.0, "Previous Gallons"=0.0, "Initial Water Level"=0.0, "Max Water Level"=0.0, "Abatements "=0, "Lid Open Events"=0, "Cycle Selected"="", "Last H Inlet "=0.0, "WOD-Detg Val Time"=0, "WOD-Total Gallons"=0, "Max Gallons"=0, "Wet Load Gallons"=0, "Gallons at EoC"=0, "Pressure at EoC"=0, "Stk Mnt Water Add"=0, "Started By remote"=FALSE, "Stopped By Remote"=FALSE, "System Reset Count"=0, "Smrt Disp at start"="", "Smrt Disp at EOC"="", "Max Jerk 1st SS"=0, "Max Jerk Final SS"=0, "Max Accelerometer"=0, "Bskt Speed Max Accel"=0, "Max Target Gallons"=0, "Jerk Delta Reject"=0, "Jerk Delta OOB "=0} ("Cycle History Diagnostics"), "Cycle End Time"=w609, "Cycles Run"=w603, "Cycle Start Time"=w597, "Cycle Knob"=w397, "Load Type"=w396, "OOB-Redistrib"=w226, "OOB-Fallbacks"=w225, "OOB-Retry"=w224, "Temp at Start"=w389, "Load Size At Start"=w388, "Deep Fill At Start"=w387, "Soil Level At Start"=w386, "Spin At Start"=w385, "Extra rinse At Start"=w582, "Deep rinse At Start"=w581, "Stain At Start"=w300, "Soak At Start"=w382, "Warm Rinse At Start"=w577, "Pauses Count"=w223, "Fault Occured"=w545, "Delay Flag"=w231, "Mycycle Flag"=w378, "Blackout"=w544, "Cycle completed"=w543, "Temp at End"=w372, "Load Size At End"=w371, "Deep Fill At End"=w370, "Soil Level At End"=w369, "Spin At End"=w368, "Extra rinse At End"=w560, "Deep rinse At End"=w559, "Stain At End"=w365, "Soak At End"=w364, "Warm Rinse At End"=w558, "Detected Load Size"=w362, "Initial Gallons"=w338, "Last C Inlet"=w346, "Last H Inlet"=w345, "Max Voltage"=w344, "Target Max Spin"=w216, "Max Spin Speed"=w217, "Initial Therm"=w343, "Max Current"=w342, "Previous Gallons"=w341, "Initial Water Level"=w340, "Max Water Level"=w339, "Abatements"=w215, "Lid Open Events"=w214, "Cycle Selected"=w347, "WOD-Detg Val Time"=w53, "WOD-Total Gallons"=w51, "Max Gallons"=w49, "Wet Load Gallons"=w27, "Gallons at EoC"=w26, "Pressure at EoC"=w25, "Stk Mnt Water Add"=w24, "Started By remote"=w23, "Stopped By Remote"=w22, "System Reset Count"=w21, "Smrt Disp at start"=w20, "Smrt Disp at EOC"=w19, "Max Jerk 1st SS"=w18, "Max Jerk Final SS"=w17, "Max Accelerometer"=w16, "Bskt Speed Max Accel"=w15, "Max Target Gallons"=w14, "Jerk Delta Reject"=w2, "Jerk Delta OOB"=w1) -> (→"output cluster":T1)
